vi "Station Detail Main.vi"(8 "error in (no error)":errorcluster, 11 "BarcodeScan in":refnum<class "BarcodeScan.lvclass">) -> (0 "error out":errorcluster, 2 "Station Out":T1=enum."ImformOut", 3 "BarcodeScan out":refnum<class "BarcodeScan.lvclass">)   [LabVIEW 2019, in "BarcodeScan.lvclass"]
uses:
  BarcodeScan.lvclass
  Ctrl/Station Action.ctl
  Ctrl/ProjectStepSelect.ctl
  Ctl/BarcodeStep.ctl
  Ctrl/Auto Inspection Station Name2.ctl
  Ctrl/Auto Inspection Data Name.ctl
  Ctl/Board Scan IO.ctl
  Ctrl/ModbusCmd.ctl
  Ctrl/Table Save.ctl
  Ctrl/MeasureDisplayTab.ctl
  LLB/Commonly VI/Main Glb.vi
  Global/Process Global.vi
  LLB/Commonly VI.lvlib
  LineScan/LineScan.lvclass
panel:
  out "Read Index Data":string
  in  "AddTable 6":string[][](table)=[["Tray Barcode", ""], ["PCBA BARCODE", ""], ["硬體(Tool初始化)", ""], ["company(Tool初始化)", ""], ["耗電流 uA(電流表)", ""], ["電池負載電壓", ""], ["晶片ID(Tool FORMAT)", ""], ["雷雕ID(TOOl scan、藍芽接收器)", ""], ["Format(Tool FORMAT)", ""], ["Programe(Tool Programe)", ""], ["MAC(藍芽接收器)", ""], ["ID(藍芽接收器)", ""], ["KPA(藍芽接收器)", ""], ["溫度(藍芽接收器)", ""], ["SENSOR電池電壓(藍芽接收器)", ""], ["RSSI(藍芽接收器)", ""], ["SensorType_315(FSK scan)", ""], ["FSKsnVol_315(FSK scan)", ""], ["FSKscanl_315(FSK scan)", ""], ["P_315(Tool FSK scan)", ""], ["T_315(Tool FSK scan)", ""], ["SensorType_433(ASK scan)", ""], ["ASKsnVol_433(ASK scan)", ""], ["ASKscan_433(ASK scan)", ""], ["P_433(ASK scan)", ""], ["T_433(ASK scan)", ""], ["測高Data", ""]]
  out "Rad In Reg":string
  in  "AddTable 2":string[][](table)=[["PCBA BARCODE", ""], ["硬體(Tool初始化)", ""], ["company(Tool初始化)", ""], ["耗電流 uA(電流表)", ""], ["電池負載電壓", ""], ["晶片ID(Tool FORMAT)", ""], ["雷雕ID(TOOl scan、藍芽接收器)", ""], ["Format(Tool FORMAT)", ""], ["Programe(Tool Programe)", ""], ["MAC(藍芽接收器)", ""], ["ID(藍芽接收器)", ""], ["KPA(藍芽接收器)", ""], ["溫度(藍芽接收器)", ""], ["SENSOR電池電壓(藍芽接收器)", ""], ["RSSI(藍芽接收器)", ""], ["SensorType_315(FSK scan)", ""], ["FSKsnVol_315(FSK scan)", ""], ["FSKscanl_315(FSK scan)", ""], ["P_315(Tool FSK scan)", ""], ["T_315(Tool FSK scan)", ""], ["SensorType_433(ASK scan)", ""], ["ASKsnVol_433(ASK scan)", ""], ["ASKscan_433(ASK scan)", ""], ["P_433(ASK scan)", ""], ["T_433(ASK scan)", ""], ["測高Data", ""]]
  out "Barcode":string
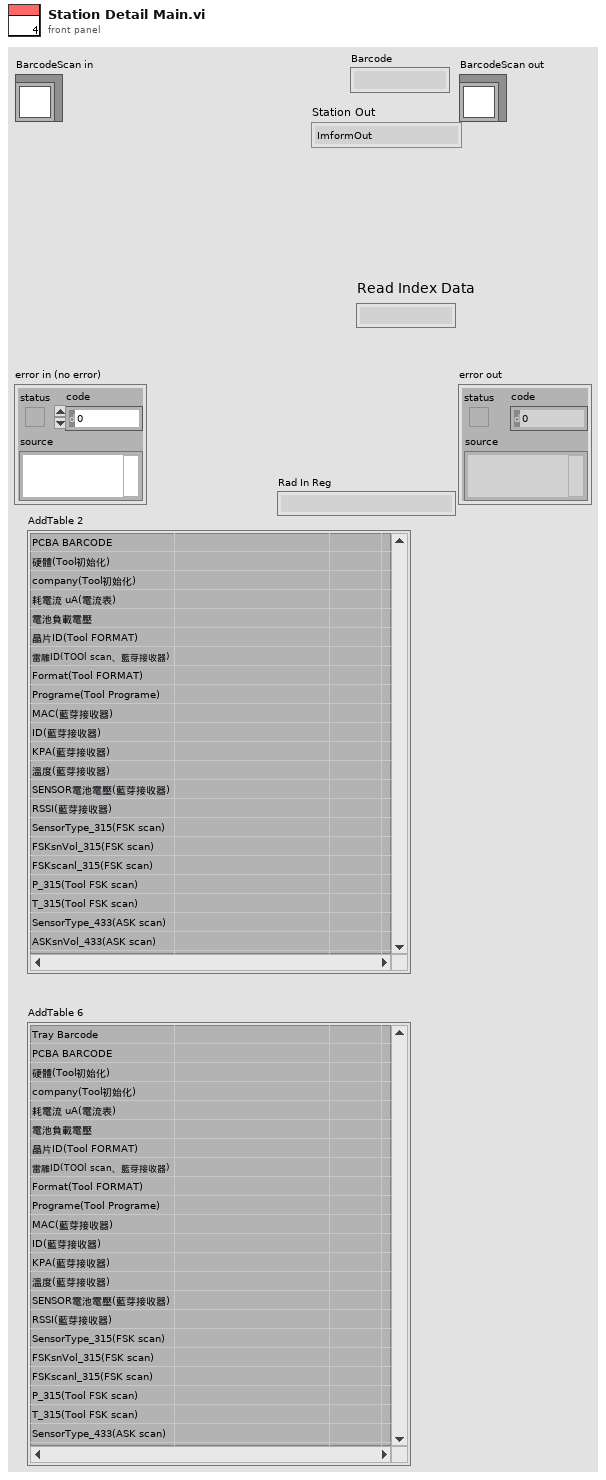
[diagram p1: front panel]
types:
  T1 = typedef "Station Action.ctl" = enum16{"Wait Item In", "Dectect Action", "ImformOut"}
  T2 = typedef "ProjectStepSelect.ctl" = enum16{"ProjectName", "Name", "Initial", "Reset", "Format", "Program1", "Program2", "Scan", "Finish", "MToolWork", "DataCheck", "DataSave", "OutputPLC", "WaitInputS1", "WaitInputOff"}
  T3 = enum16{"initial", "Add", "Write", "Replace", "Delete", "REad"}
  T4 = typedef "Auto Inspection Data Name.ctl" = enum16{"LocalRun", "ItemSN(TimeCode)", "CurrentAction", "Error", "Data", "OKNG", "電壓值", "電壓值判斷", "電流值", "電流值判斷", "Laser1 Data", "Laser2 Data", "Laser OKNG", "StationNO"}
  T5 = typedef "Auto Inspection Station Name2.ctl" = enum16{"S1Barcode", "S2Measure", "S3Measure", "S4Measure", "S5Measure", "S11_LaserCheck", "S8_Vision AI"}
  T6 = cluster{"starting address":u16, "number of inputs":u16, "Sat Coils":bool[], "Holding Registers":u16[]}
  T7 = typedef "ModbusCmd.ctl" = enum16{"Connect", "Disconnect", "Init", "Fetch Basic Objects", "Fetch Input Refisters", "Fetch Discrete Inputs", "Set Coils", "Set Holding Registers", "Write Single Holding", "Exit"}
  T8 = typedef "BarcodeStep.ctl" = enum16{"Initial", "BarcodeScan", "BcdCheck", "BcdCheckOK", "ReadPLCBarcode", "BcdCheckNG", "Merge", "SendPLC_OK", "DataSave", "IOSignal Off", "Finish"}
  T9 = enum16{"載盤條碼比對需求", "載盤條碼比對OK", "載盤條碼比對NG", "S1可讀取訊號"}
  T10 = typedef "Board Scan IO.ctl" = enum16{"S1 Barcode Scan", "回給PLC完成讀取訊號", "S1 載盤條碼比對NG", "S1PLC 條碼可讀取訊號", "S1備用_04", "S1備用_05", "S1備用_06", "S1備用_07", "S1備用_08", "S1 發送條碼完成"}
  T11 = typedef "MeasureDisplayTab.ctl" = enum16{"Tray Barcode", "PCBA BARCODE", "硬體(Tool初始化)", "company(Tool初始化)", "耗電流 uA(電流表)", "電池負載電壓", "晶片ID(Tool FORMAT)", "雷雕ID(TOOl scan、藍芽接收器)", "Format(Tool FORMAT)", "Programe(Tool Programe)", "MAC(藍芽接收器)", "ID(藍芽接收器)", "KPA(藍芽接收器)", "溫度(藍芽接收器)", "SENSOR電池電壓(藍芽接收器)", "RSSI(藍芽接收器)", "SensorType_315(FSK scan)", "FSKsnVol_315(FSK scan)", "FSKscanl_315(FSK scan)", "P_315(FSK scan)", "T_315(FSK scan)", "SensorType_433(ASK scan)", "ASKsnVol_433(ASK scan)", "ASKscan_433(ASK scan)", "P_433(ASK scan)", "T_433(ASK scan)", "測高Data"}
  T12 = typedef "Table Save.ctl" = enum16{"initial", "Add", "Write", "Replace", "Delete", "REad", "RedTable", "Load"}
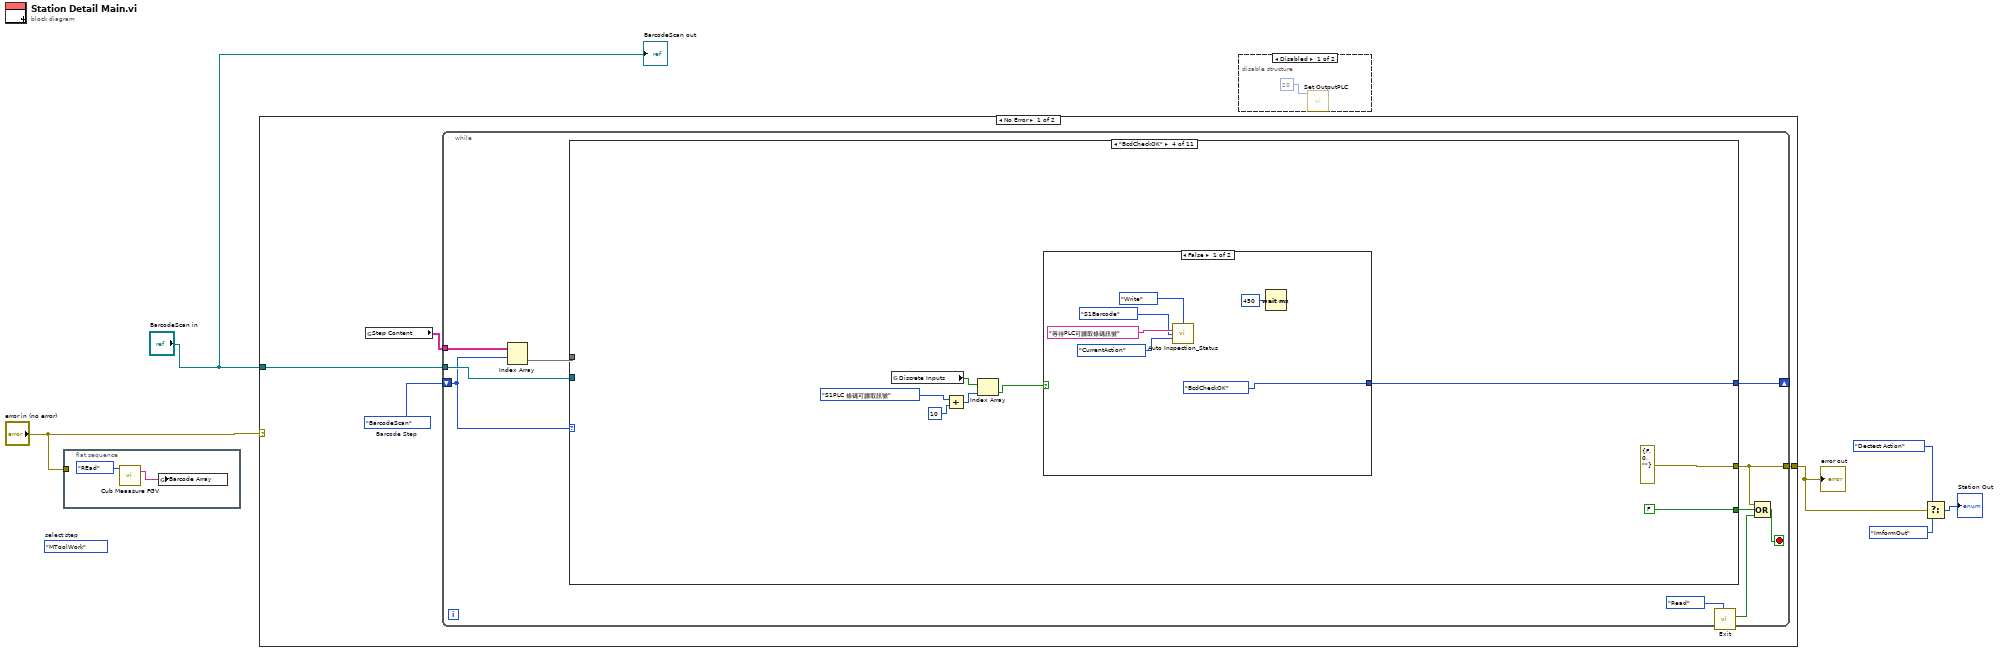
[diagram p0: block diagram]
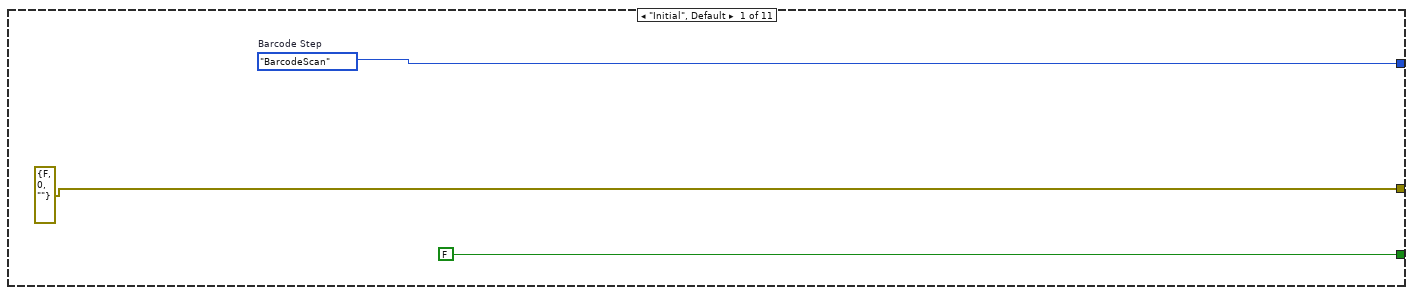
[diagram p3: hidden frame]
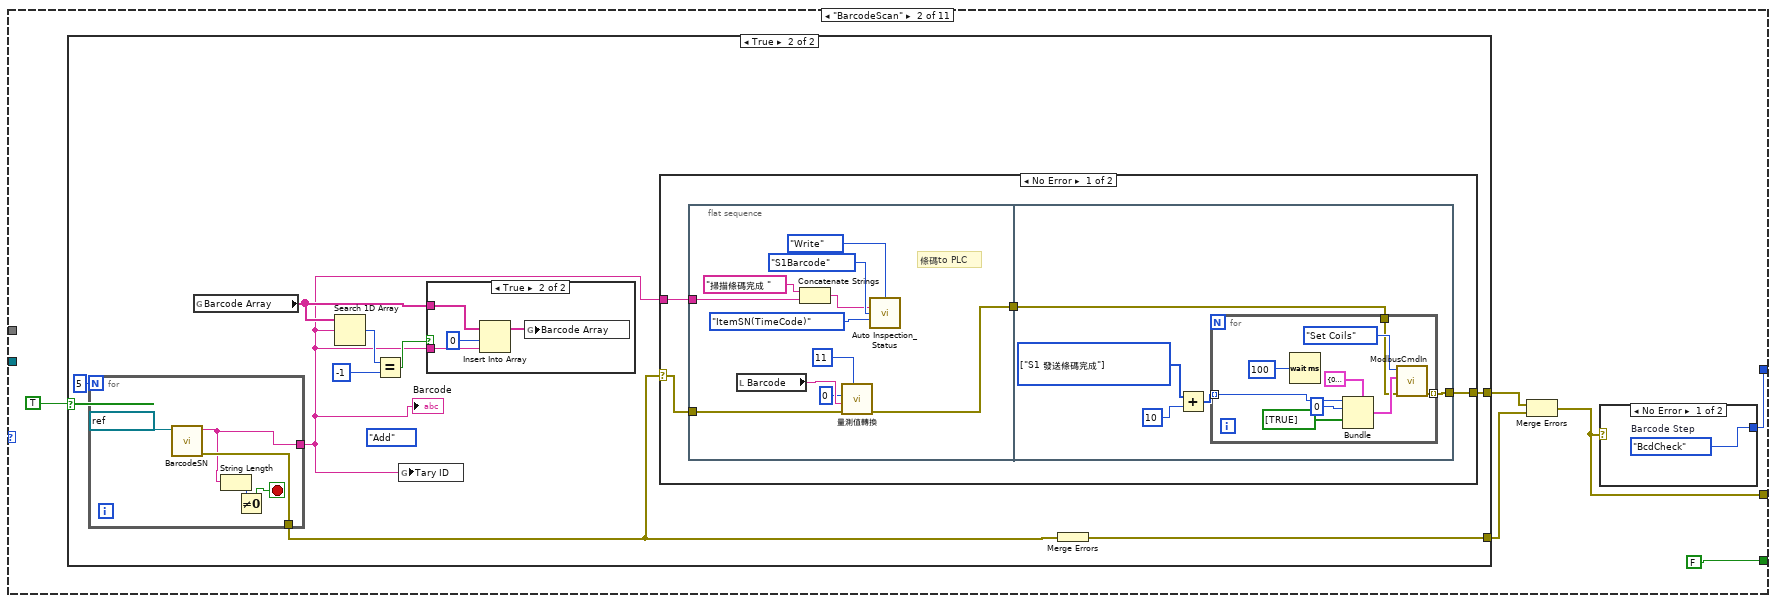
[diagram p4: hidden frame]
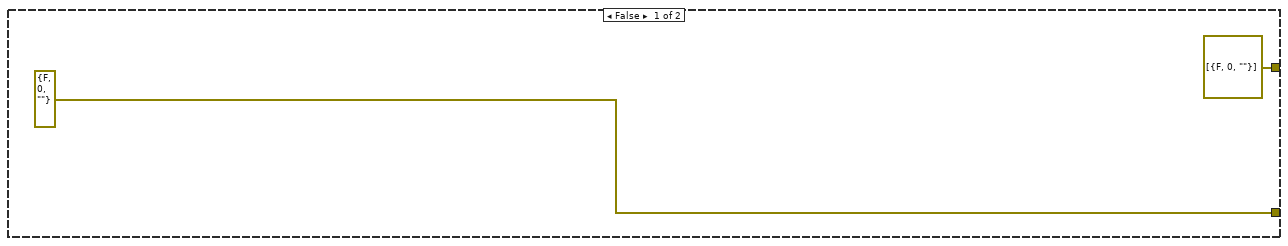
[diagram p5: hidden frame]
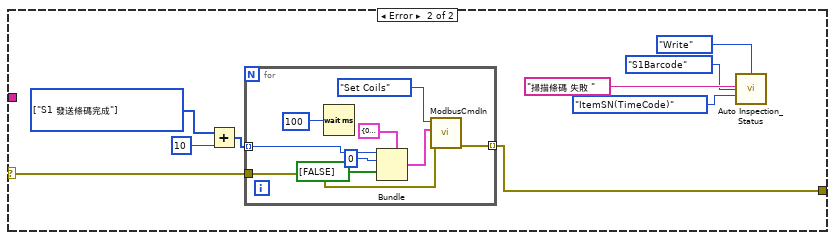
[diagram p6: hidden frame]
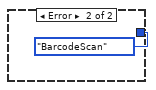
[diagram p8: hidden frame]
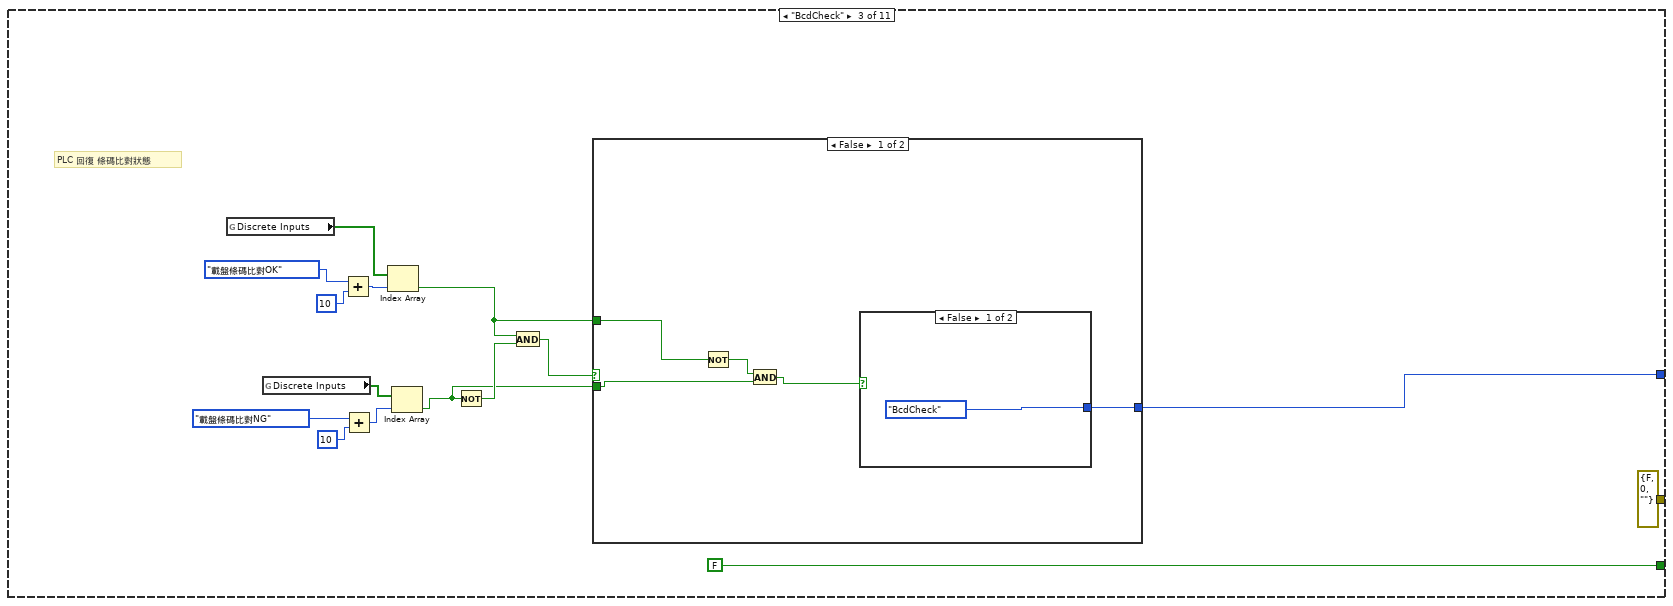
[diagram p9: hidden frame]
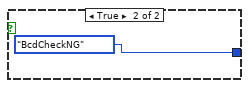
[diagram p10: hidden frame]
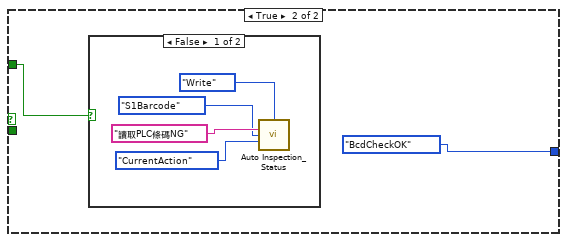
[diagram p11: hidden frame]
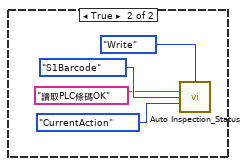
[diagram p12: hidden frame]
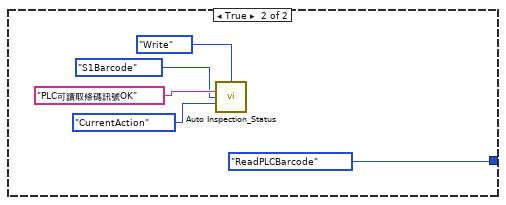
[diagram p13: hidden frame]
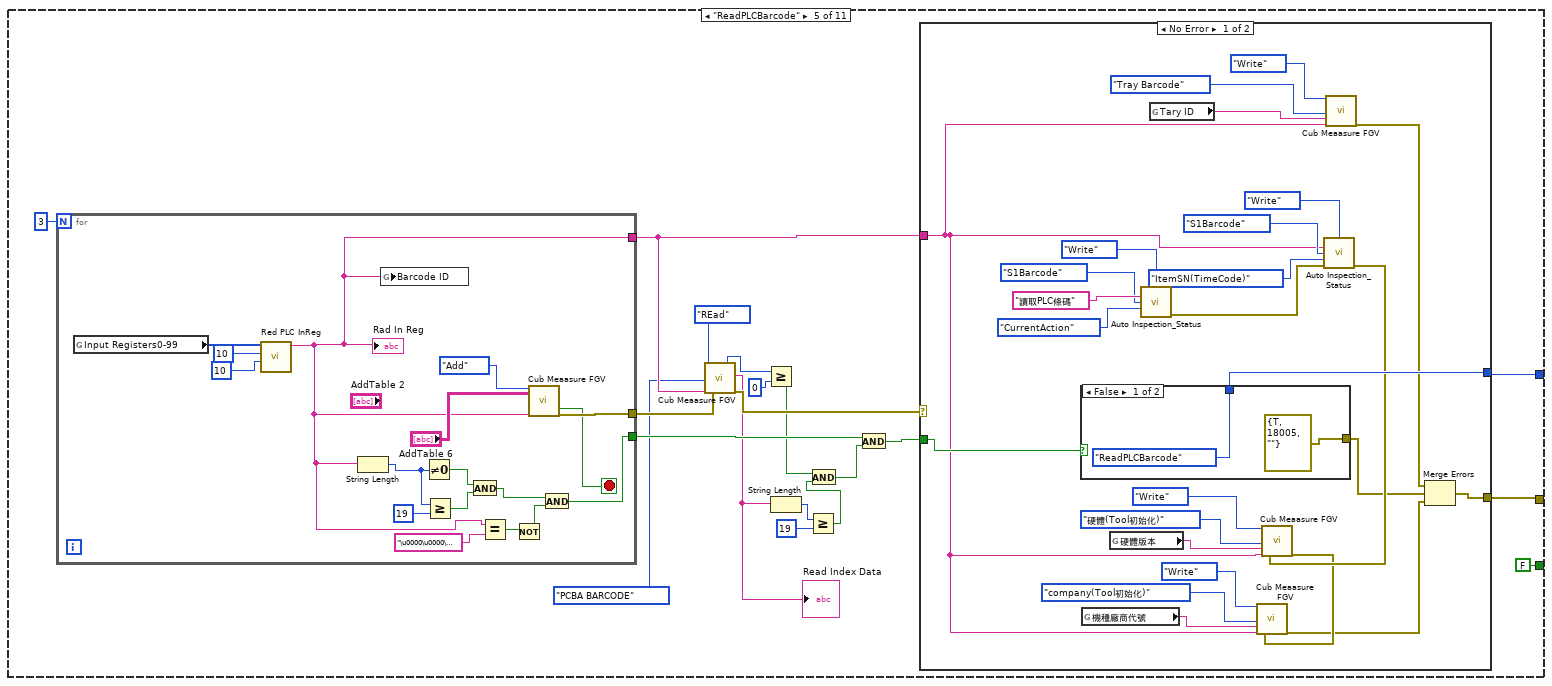
[diagram p14: hidden frame]
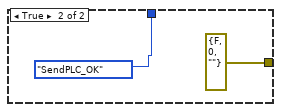
[diagram p15: hidden frame]
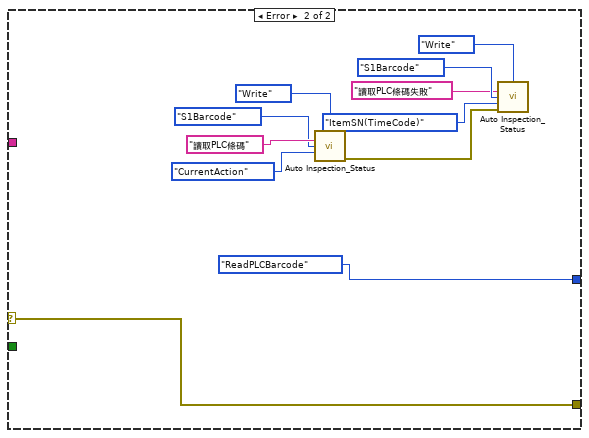
[diagram p16: hidden frame]
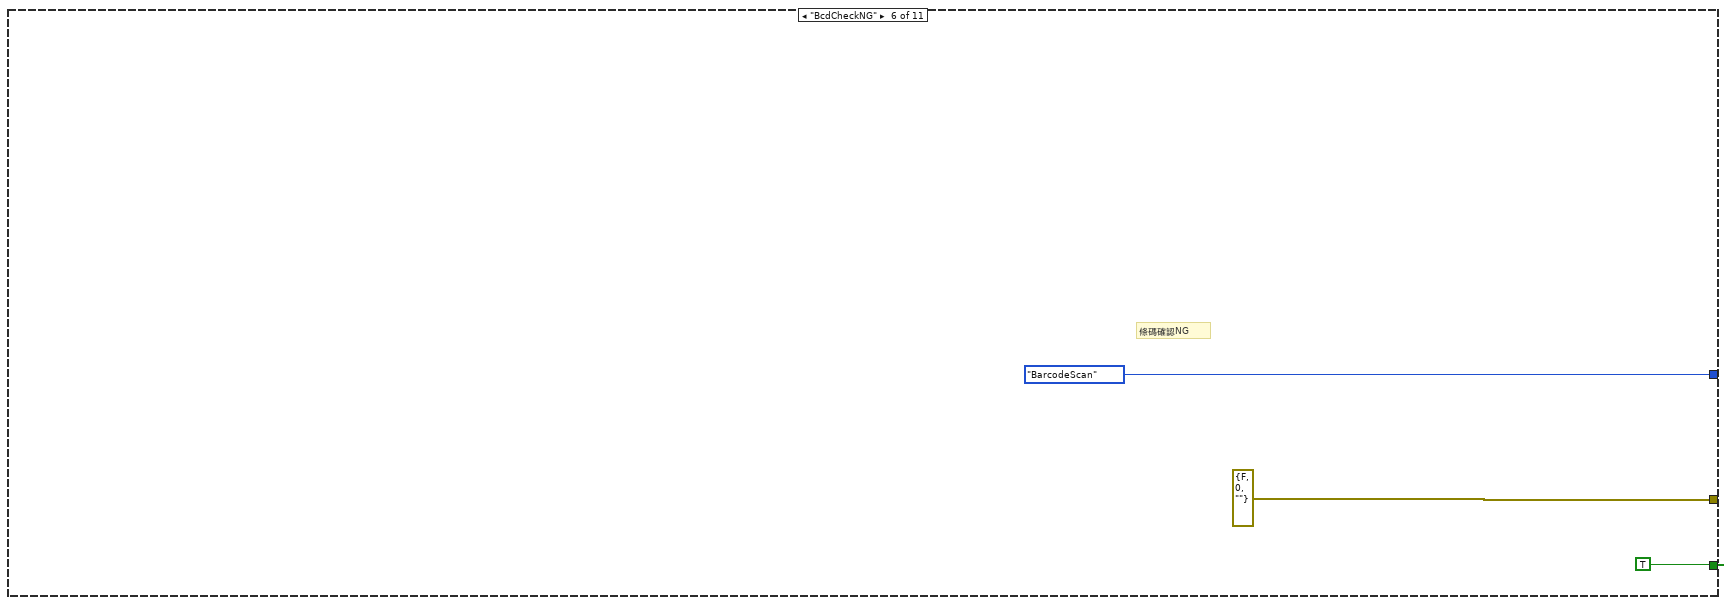
[diagram p17: hidden frame]
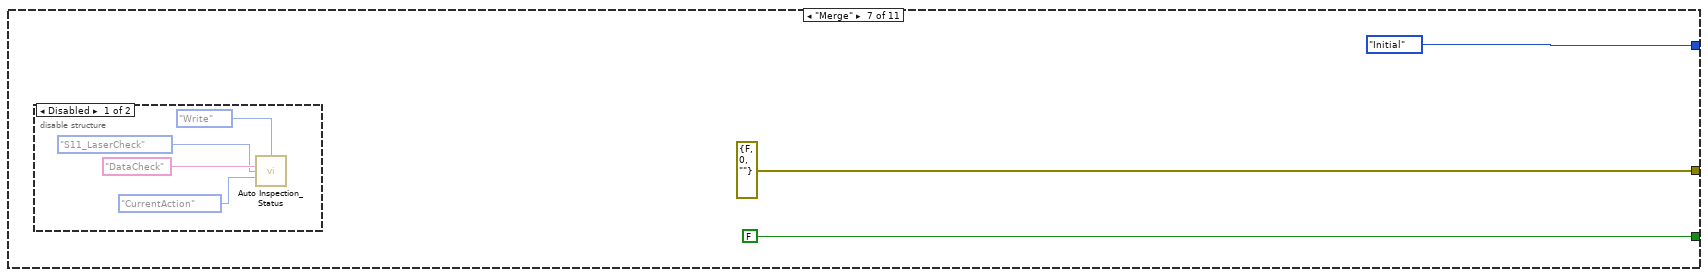
[diagram p18: hidden frame]
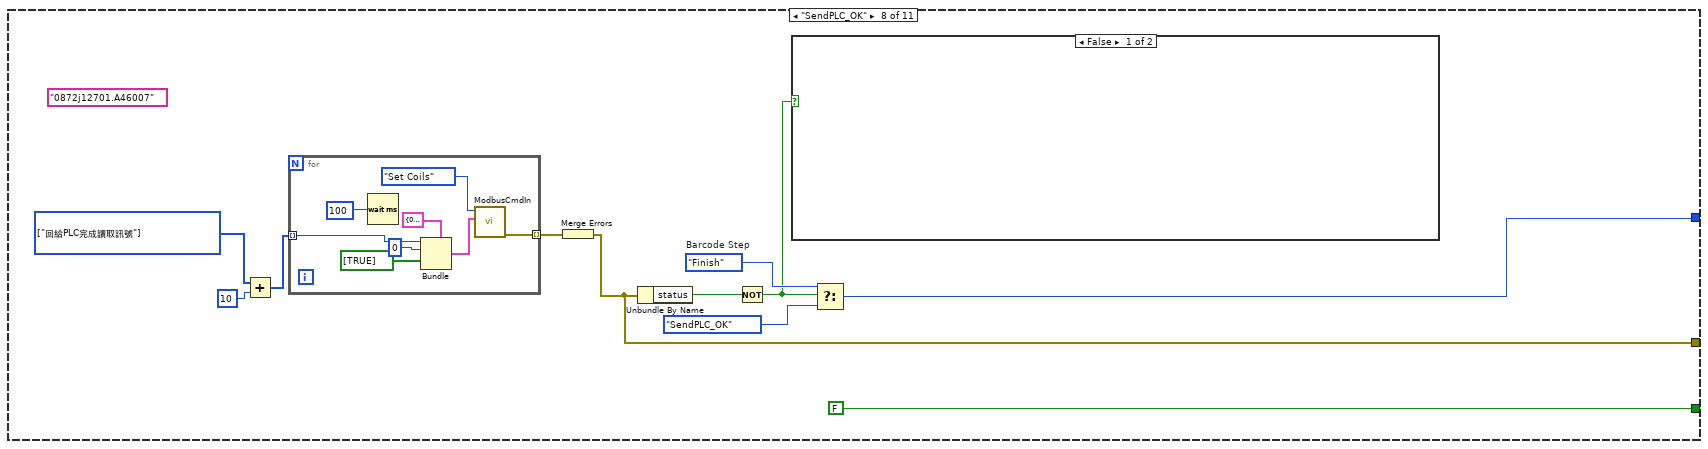
[diagram p20: hidden frame]
diagram:
  (unwired) ProjectStepSelect."MToolWork"  # select step
  n1 = flat-sequence {
    tunnel: "error in (no error)" -> [_]
    frame #0 {
      n2 = call "Cub Meaasure FGV.vi"("Action"=T3."REad" ("Enum")) -> ("Barcode Array"=w8:string[])  [unwired: 11 in, 7 out]
      n3 = global write "Main Glb.vi" "Barcode Array"(w8) -> ()
    }
  }
  n4 = case shown="No Error" "error in (no error)" {
    selector: "error in (no error)" -> [_ w288]
    tunnel: [w12 w288] -> w3
    tunnel: "BarcodeScan in" -> [w11 _]
    frame No Error {
      w9 = BarcodeStep."BarcodeScan"  # Barcode Step
      n5 = global read "Process Global.vi" "Step Content"() -> (w10:string[][])
      n6 = while {
        tunnel: [w17] -> w12
        shift-right: [w22] -> _
        shift-left: w9 -> [w18]
        tunnel: w11 -> [w19]
        tunnel: w10 -> [w20]
        stop <- w16 stop-if-true
        n7 = Index Array(array=w20, index (row)=w18) -> (element=w21:string[])  [unwired: 1 in]
        n8 = case shown="\"BcdCheckOK\"" w18 {
          tunnel: [errorcluster {"status"=FALSE, "code"=0, "source"=""} ("error constant") w26 errorcluster {"status"=FALSE, "code"=0, "source"=""} ("error IO") errorcluster {"status"=FALSE, "code"=0, "source"=""} ("error IO") w169 errorcluster {"status"=FALSE, "code"=0, "source"=""} ("error IO") errorcluster {"status"=FALSE, "code"=0, "source"=""} ("error IO") w239 w259 w267 errorcluster {"status"=FALSE, "code"=0, "source"=""} ("error IO")] -> w17
          tunnel: [w23 w29 w107 w136 w170 BarcodeStep."BarcodeScan" ("Barcode Step") BarcodeStep."Initial" ("Barcode Step") w246 BarcodeStep."IOSignal Off" ("Barcode Step") w268 w285] -> w22
          tunnel: w19 -> [_ _ _ _ _ _ _ _ _ _ _]
          tunnel: w21 -> [_ _ _ _ _ _ _ _ _ _ _]
          tunnel: [FALSE FALSE FALSE FALSE FALSE TRUE FALSE FALSE FALSE FALSE TRUE] -> w15
          frame "Initial", Default {
            w23 = BarcodeStep."BarcodeScan"  # Barcode Step
          }
          frame "BarcodeScan" {
            n9 = case shown="True" TRUE {
              tunnel: [errorcluster {"status"=FALSE, "code"=0, "source"=""} ("error out") w38] -> w27
              tunnel: [errorcluster[] [{"status"=FALSE, "code"=0, "source"=""}] w36] -> w28
              frame False {
              }
              frame True {
                (unwired) T3."Add" ("Enum")
                n10 = for {
                  N: 5 -> [_]
                  tunnel: [w46] -> w37
                  tunnel: [w45] -> w35
                  stop <- w44 stop-if-true
                  n11 = call "BarcodeSN.vi"("VISA resource name"=refnum<visa-resource-name> "COM9") -> ("error out"=w46:errorcluster, "Barcode"=w45:string)  [unwired: 9 in]
                  n12 = String Length(string=w45) -> (length=w43:i32)
                  n13 = Not Equal To 0?(x=w43) -> (x != 0?=w44:bool)
                }
                "Barcode" <- w35
                n14 = global read "Main Glb.vi" "Barcode Array"() -> (w41:string[])
                n15 = Search 1D Array(1D array=w41, element=w35) -> (index of element=w40:i32)  [unwired: 1 in]
                n16 = Equal?(x=w40, y=-1) -> (x = y?=w42:bool)
                n17 = global write "Main Glb.vi" "Tary ID"(w35) -> ()
                n18 = case shown="True" w42 {
                  tunnel: w41 -> [_ w98]
                  tunnel: w35 -> [_ w97]
                  frame False {
                  }
                  frame True {
                    n19 = Insert Into Array(array=w98, index=0, new element=w97) -> (w95:string[])
                    n20 = global write "Main Glb.vi" "Barcode Array"(w95) -> ()
                  }
                }
                n21 = case shown="No Error" w37 {
                  selector: w37 -> [w51 w81]
                  tunnel: [w49 w80] -> w36
                  tunnel: w35 -> [w48 _]
                  frame No Error {
                    n22 = flat-sequence {
                      tunnel: w51 -> [w56]
                      tunnel: [w55] -> w50
                      tunnel: w48 -> [w53]
                      tunnel: w50 -> [w67]
                      tunnel: [w66] -> w49
                      frame #0 {
                        # "條碼to PLC"
                        n23 = local read "Barcode"() -> (w59:string)
                        n24 = Concatenate Strings("掃描條碼完成 " ("DataIn"), w53) -> (w52:string)
                        n25 = call "量測值轉換.vi"("位數"=11, "error in (no error)"=w56, "input string"=w59, "PLC address"=0) -> ("error out"=w55:errorcluster)  [unwired: 6 in, 1 out]
                        n26 = call "Auto Inspection_Status.vi"("Action"=enum16{"Initial", "Write", "Read"}."Write", "DataIn"=w52, "Station"=Auto_Inspection_Station_Name2."S1Barcode", "Data"=Auto_Inspection_Data_Name."ItemSN(TimeCode)") -> ()  [unwired: 9 in, 3 out]
                      }
                      frame #1 {
                        w65 = T10[] [enum."S1 發送條碼完成"] items=["S1 Barcode Scan", "回給PLC完成讀取訊號", "S1 載盤條碼比對NG", "S1PLC 條碼可讀取訊號", "S1備用_04", "S1備用_05", "S1備用_06", "S1備用_07", "S1備用_08", "S1 發送條碼完成"]
                        n27 = Add(x=w65, y=10) -> (x+y=w63:i32[])
                        n28 = for {
                          tunnel: [w70] -> w66 mode=indexing
                          tunnel: w63 -> [w69] mode=indexing
                          tunnel: w67 -> [w68]
                          n29 = Wait (ms)(milliseconds to wait=100) -> ()  [unwired: 1 out]
                          n30 = Bundle(cluster=T6 {"starting address"=0, "number of inputs"=0, "Sat Coils"=[], "Holding Registers"=[]} ("data"), "starting address"=w69, "number of inputs"=u16 0, "Sat Coils"=bool[] [TRUE]) -> (w73:T6)  [unwired: 1 in]
                          n31 = call "ModbusCmdIn.vi"("error in (no error)"=w68, "data"=w73, "Enum"=ModbusCmd."Set Coils") -> ("error out"=w70:errorcluster)  [unwired: 8 in]
                        }
                      }
                    }
                  }
                  frame Error {
                    w79 = T10[] [enum."S1 發送條碼完成"] items=["S1 Barcode Scan", "回給PLC完成讀取訊號", "S1 載盤條碼比對NG", "S1PLC 條碼可讀取訊號", "S1備用_04", "S1備用_05", "S1備用_06", "S1備用_07", "S1備用_08", "S1 發送條碼完成"]
                    n32 = Add(x=w79, y=10) -> (x+y=w77:i32[])
                    n33 = for {
                      tunnel: [w88] -> w80 mode=indexing
                      tunnel: w77 -> [w87] mode=indexing
                      tunnel: w81 -> [w86]
                      n34 = Wait (ms)(milliseconds to wait=100) -> ()  [unwired: 1 out]
                      n35 = Bundle(cluster=T6 {"starting address"=0, "number of inputs"=0, "Sat Coils"=[], "Holding Registers"=[]} ("data"), "starting address"=w87, "number of inputs"=u16 0, "Sat Coils"=bool[] [FALSE]) -> (w91:T6)  [unwired: 1 in]
                      n36 = call "ModbusCmdIn.vi"("error in (no error)"=w86, "data"=w91, "Enum"=ModbusCmd."Set Coils") -> ("error out"=w88:errorcluster)  [unwired: 8 in]
                    }
                    n37 = call "Auto Inspection_Status.vi"("Action"=enum16{"Initial", "Write", "Read"}."Write", "DataIn"="掃描條碼 失敗 ", "Station"=Auto_Inspection_Station_Name2."S1Barcode", "Data"=Auto_Inspection_Data_Name."ItemSN(TimeCode)") -> ()  [unwired: 9 in, 3 out]
                  }
                }
                n38 = Merge Errors(w37) -> (w38:errorcluster)
              }
            }
            n39 = Merge Errors(w28, w27) -> (w26:errorcluster)
            n40 = case shown="No Error" w26 {
              tunnel: [w99 BarcodeStep."BarcodeScan" ("Barcode Step")] -> w29
              frame No Error {
                w99 = BarcodeStep."BcdCheck"  # Barcode Step
              }
              frame Error {
              }
            }
          }
          frame "BcdCheck" {
            # "PLC 回復 條碼比對狀態"
            n41 = global read "Main Glb.vi" "Discrete Inputs"() -> (w114:bool[])
            n42 = global read "Main Glb.vi" "Discrete Inputs"() -> (w109:bool[])
            n43 = Add(x=T9."載盤條碼比對OK", y=10) -> (x+y=w112:i32)
            n44 = Add(x=T9."載盤條碼比對NG", y=10) -> (x+y=w111:i32)
            n45 = Index Array(array=w114, index=w112) -> (element=w105:bool)
            n46 = Index Array(array=w109, index=w111) -> (element=w104:bool)
            n47 = Not(x=w104) -> (.not. x?=w108:bool)
            n48 = And(x=w105, y=w108) -> (x .and. y?=w106:bool)
            n49 = case shown="False" w106 {
              tunnel: [w116 BarcodeStep."BcdCheckOK" ("Barcode Step")] -> w107
              tunnel: w105 -> [w120 w123]
              tunnel: w104 -> [w118 _]
              frame False {
                n50 = Not(x=w120) -> (.not. x?=w119:bool)
                n51 = And(x=w119, y=w118) -> (x .and. y?=w117:bool)
                n52 = case shown="False" w117 {
                  tunnel: [BarcodeStep."BcdCheck" ("Barcode Step") BarcodeStep."BcdCheckNG" ("Barcode Step")] -> w116
                  frame False {
                  }
                  frame True {
                  }
                }
              }
              frame True {
                n53 = case shown="False" w123 {
                  frame False {
                    n54 = call "Auto Inspection_Status.vi"("Action"=enum16{"Initial", "Write", "Read"}."Write", "DataIn"="讀取PLC條碼NG", "Station"=Auto_Inspection_Station_Name2."S1Barcode", "Data"=Auto_Inspection_Data_Name."CurrentAction") -> ()  [unwired: 9 in, 3 out]
                  }
                  frame True {
                    n55 = call "Auto Inspection_Status.vi"("Action"=enum16{"Initial", "Write", "Read"}."Write", "DataIn"="讀取PLC條碼OK", "Station"=Auto_Inspection_Station_Name2."S1Barcode", "Data"=Auto_Inspection_Data_Name."CurrentAction") -> ()  [unwired: 9 in, 3 out]
                  }
                }
              }
            }
          }
          frame "BcdCheckOK" {
            n56 = global read "Main Glb.vi" "Discrete Inputs"() -> (w140:bool[])
            n57 = Add(x=Board_Scan_IO."S1PLC 條碼可讀取訊號" ("Enum"), y=10) -> (x+y=w138:i32)
            n58 = Index Array(array=w140, index=w138) -> (element=w135:bool)
            n59 = case shown="False" w135 {
              tunnel: [BarcodeStep."BcdCheckOK" ("Barcode Step") BarcodeStep."ReadPLCBarcode" ("Barcode Step")] -> w136
              frame False {
                n60 = call "Auto Inspection_Status.vi"("Action"=enum16{"Initial", "Write", "Read"}."Write", "DataIn"="等待PLC可讀取條碼訊號", "Station"=Auto_Inspection_Station_Name2."S1Barcode", "Data"=Auto_Inspection_Data_Name."CurrentAction") -> ()  [unwired: 9 in, 3 out]
                n61 = Wait (ms)(milliseconds to wait=u32 450) -> ()  [unwired: 1 out]
              }
              frame True {
                n62 = call "Auto Inspection_Status.vi"("Action"=enum16{"Initial", "Write", "Read"}."Write", "DataIn"="PLC可讀取條碼訊號OK", "Station"=Auto_Inspection_Station_Name2."S1Barcode", "Data"=Auto_Inspection_Data_Name."CurrentAction") -> ()  [unwired: 9 in, 3 out]
              }
            }
          }
          frame "ReadPLCBarcode" {
            n63 = for {
              N: 3 -> [_]
              tunnel: [w171] -> w166
              tunnel: [w183] -> w160
              tunnel: [w176] -> w165
              stop <- w182 stop-if-true
              n64 = global read "Main Glb.vi" "Input Registers0-99"() -> (w187:u16[])
              n65 = call "Red PLC InReg.vi"("length"=10, "index"=10, "Input Registers Arr"=w187) -> ("Rad In Reg"=w176:string)  [unwired: 7 in, 1 out]
              "Rad In Reg" <- w176
              n66 = String Length(string=w176) -> (length=w180:i32)
              n67 = global write "Main Glb.vi" "Barcode ID"(w176) -> ()
              n68 = Not Equal To 0?(x=w180) -> (x != 0?=w178:bool)
              n69 = Greater Or Equal?(x=w180, y=19) -> (x >= y?=w177:bool)
              n70 = And(x=w178, y=w177) -> (x .and. y?=w172:bool)
              n71 = Equal?(x=w176, y="\u0000\u0000\u0000\u0000\u0000\u0000\u0000\u0000\u0000\u0000\u0000\u0000\u0000\u0000\u0000\u0000\u0000\u0000\u0000\u0000") -> (x = y?=w174:bool)
              n72 = Not(x=w174) -> (.not. x?=w173:bool)
              n73 = call "Cub Meaasure FGV.vi"("Action"=T3."Add" ("Enum"), "AddTable 6"="AddTable 6", "SN"=w176) -> ("Barcode重複"=w182:bool, "error out"=w183:errorcluster)  [unwired: 9 in, 6 out]
              n74 = And(x=w172, y=w173) -> (x .and. y?=w171:bool)
            }
            n75 = call "Cub Meaasure FGV.vi"("Action"=Table_Save."REad", "Save Index"=MeasureDisplayTab."PCBA BARCODE", "SN"=w165, "error in (no error)"=w160) -> ("條碼的Index"=w163:i32, "Read Index Data"=w155:string, "error out"=w159:errorcluster)  [unwired: 8 in, 5 out]
            "Read Index Data" <- w155
            n76 = Greater Or Equal?(x=w163, y=0) -> (x >= y?=w157:bool)
            n77 = String Length(string=w155) -> (length=w154:i32)
            n78 = Greater Or Equal?(x=w154, y=19) -> (x >= y?=w152:bool)
            n79 = And(x=w157, y=w152) -> (x .and. y?=w156:bool)
            n80 = And(x=w166, y=w156) -> (x .and. y?=w161:bool)
            n81 = case shown="No Error" w159 {
              selector: w159 -> [_ w227]
              tunnel: [w213 BarcodeStep."ReadPLCBarcode" ("Enum")] -> w170
              tunnel: w161 -> [w204 _]
              tunnel: [w193 w227] -> w169
              tunnel: w165 -> [w190 _]
              frame No Error {
                n82 = case shown="False" w204 {
                  tunnel: [BarcodeStep."ReadPLCBarcode" ("Enum") BarcodeStep."SendPLC_OK" ("Enum")] -> w213
                  tunnel: [errorcluster {"status"=TRUE, "code"=18005, "source"=""} ("error IO") errorcluster {"status"=FALSE, "code"=0, "source"=""} ("error IO")] -> w194
                  frame False {
                  }
                  frame True {
                  }
                }
                n83 = global read "Process Global.vi" "機種廠商代號"() -> (w198:string)
                n84 = global read "Process Global.vi" "硬體版本"() -> (w199:string)
                n85 = call "Auto Inspection_Status.vi"("Action"=enum16{"Initial", "Write", "Read"}."Write", "DataIn"="讀取PLC條碼", "Station"=Auto_Inspection_Station_Name2."S1Barcode", "Data"=Auto_Inspection_Data_Name."CurrentAction") -> ("error out"=w205:errorcluster)  [unwired: 9 in, 2 out]
                n86 = global read "Main Glb.vi" "Tary ID"() -> (w189:string)
                n87 = call "Auto Inspection_Status.vi"("Action"=enum16{"Initial", "Write", "Read"}."Write", "DataIn"=w190, "Station"=Auto_Inspection_Station_Name2."S1Barcode", "Data"=Auto_Inspection_Data_Name."ItemSN(TimeCode)", "error in"=w205) -> ("error out"=w197:errorcluster)  [unwired: 8 in, 2 out]
                n88 = call "Cub Meaasure FGV.vi"("Action"=Table_Save."Write" ("Enum"), "Save Index"=MeasureDisplayTab."硬體(Tool初始化)", "DataIn"=w199, "SN"=w190, "error in (no error)"=w197) -> ("error out"=w196:errorcluster)  [unwired: 7 in, 7 out]
                n89 = call "Cub Meaasure FGV.vi"("Action"=Table_Save."Write" ("Enum"), "Save Index"=MeasureDisplayTab."company(Tool初始化)", "DataIn"=w198, "SN"=w190, "error in (no error)"=w196) -> ("error out"=w195:errorcluster)  [unwired: 7 in, 7 out]
                n90 = call "Cub Meaasure FGV.vi"("Action"=Table_Save."Write" ("Enum"), "Save Index"=MeasureDisplayTab."Tray Barcode", "DataIn"=w189, "SN"=w190) -> ("error out"=w188:errorcluster)  [unwired: 8 in, 7 out]
                n91 = Merge Errors(w188, w194, w195) -> (w193:errorcluster)
              }
              frame Error {
                n92 = call "Auto Inspection_Status.vi"("Action"=enum16{"Initial", "Write", "Read"}."Write", "DataIn"="讀取PLC條碼", "Station"=Auto_Inspection_Station_Name2."S1Barcode", "Data"=Auto_Inspection_Data_Name."CurrentAction") -> ("error out"=w219:errorcluster)  [unwired: 9 in, 2 out]
                n93 = call "Auto Inspection_Status.vi"("Action"=enum16{"Initial", "Write", "Read"}."Write", "DataIn"="讀取PLC條碼失敗", "Station"=Auto_Inspection_Station_Name2."S1Barcode", "Data"=Auto_Inspection_Data_Name."ItemSN(TimeCode)", "error in"=w219) -> ()  [unwired: 8 in, 3 out]
              }
            }
          }
          frame "BcdCheckNG" {
            # "條碼確認NG"
          }
          frame "Merge" {
            n94 = disable-structure shown="Disabled" {
              frame Disabled {
                n95 = call "Auto Inspection_Status.vi"("Action"=enum16{"Initial", "Write", "Read"}."Write", "DataIn"="DataCheck", "Station"=Auto_Inspection_Station_Name2."S11_LaserCheck", "Data"=Auto_Inspection_Data_Name."CurrentAction") -> ()  [unwired: 9 in, 3 out]
              }
              frame Enabled {
              }
            }
          }
          frame "SendPLC_OK" {
            w242 = T10[] [enum."回給PLC完成讀取訊號"] items=["S1 Barcode Scan", "回給PLC完成讀取訊號", "S1 載盤條碼比對NG", "S1PLC 條碼可讀取訊號", "S1備用_04", "S1備用_05", "S1備用_06", "S1備用_07", "S1備用_08", "S1 發送條碼完成"]
            w247 = BarcodeStep."Finish"  # Barcode Step
            (unwired) "0872j12701.A46007" ("String Input")
            n96 = Add(x=w242, y=10) -> (x+y=w241:i32[])
            n97 = for {
              tunnel: [w251] -> w240 mode=indexing
              tunnel: w241 -> [w250] mode=indexing
              n98 = Wait (ms)(milliseconds to wait=100) -> ()  [unwired: 1 out]
              n99 = Bundle(cluster=T6 {"starting address"=0, "number of inputs"=0, "Sat Coils"=[], "Holding Registers"=[]} ("data"), "starting address"=w250, "number of inputs"=u16 0, "Sat Coils"=bool[] [TRUE]) -> (w254:T6)  [unwired: 1 in]
              n100 = call "ModbusCmdIn.vi"("data"=w254, "Enum"=ModbusCmd."Set Coils") -> ("error out"=w251:errorcluster)  [unwired: 9 in]
            }
            n101 = Merge Errors(w240) -> (w239:errorcluster)
            n102 = Unbundle By Name(w239) -> ("status"=w248:bool)
            n103 = Not(x=w248) -> (.not. x?=w245:bool)
            n104 = case shown="False" w245 {
              frame False {
              }
              frame True {
              }
            }
            n105 = Select(t=w247, s=w245, f=BarcodeStep."SendPLC_OK" ("Barcode Step")) -> (s? t:f=w246:T8)
          }
          frame "DataSave" {
            # "給PLC訊號"
            n106 = disable-structure shown="Enabled" {
              disable-tunnel: [_ errorcluster {"status"=FALSE, "code"=0, "source"=""} ("error IO")] -> w259
              frame Disabled {
              }
              frame Enabled {
                n107 = local read "Barcode"() -> (w261:string)
                n108 = call "Auto Inspection_Status.vi"("Action"=enum16{"Initial", "Write", "Read"}."Write", "DataIn"=w261, "Station"=Auto_Inspection_Station_Name2."S1Barcode", "Data"=Auto_Inspection_Data_Name."ItemSN(TimeCode)") -> ()  [unwired: 9 in, 3 out]
              }
            }
          }
          frame "IOSignal Off" {
            w274 = T10[] [enum."S1 Barcode Scan"] items=["S1 Barcode Scan", "回給PLC完成讀取訊號", "S1 載盤條碼比對NG", "S1PLC 條碼可讀取訊號", "S1備用_04", "S1備用_05", "S1備用_06", "S1備用_07", "S1備用_08", "S1 發送條碼完成"]
            # "條碼掃描完成"
            n109 = for {
              tunnel: w274 -> [w277] mode=indexing
              tunnel: [w275] -> w273 mode=indexing
              n110 = Wait (ms)(milliseconds to wait=100) -> ()  [unwired: 1 out]
              n111 = Add(x=w277, y=u16 10 ("starting address")) -> (x+y=w284:u16)
              n112 = Bundle(cluster=T6 {"starting address"=0, "number of inputs"=0, "Sat Coils"=[], "Holding Registers"=[]} ("data"), "starting address"=w284, "number of inputs"=u16 0, "Sat Coils"=bool[] [FALSE]) -> (w279:T6)  [unwired: 1 in]
              n113 = call "ModbusCmdIn.vi"("data"=w279, "Enum"=ModbusCmd."Set Coils") -> ("error out"=w275:errorcluster)  [unwired: 9 in]
            }
            n114 = Merge Errors(w273) -> (w267:errorcluster)
            n115 = Unbundle By Name(w267) -> ("status"=w272:bool)
            n116 = Not(x=w272) -> (.not. x?=w271:bool)
            n117 = Select(t=BarcodeStep."Finish" ("Barcode Step"), s=w271, f=BarcodeStep."IOSignal Off" ("Barcode Step")) -> (s? t:f=w268:T8)
          }
          frame "Finish" {
            w285 = BarcodeStep."BarcodeScan"  # Barcode Step
          }
        }
        n118 = call "Exit.vi"("Enum"=enum16{"Initial", "Read", "Write"}."Read") -> ("ExitOut"=w14:bool)  [unwired: 10 in]
        n119 = Compound Arithmetic op=OR(w17, w15, w14) -> (w16:bool)
      }
    }
    frame Error {
    }
  }
  "error out" <- w3
  n120 = disable-structure shown="Disabled" {
    frame Disabled {
      n121 = call "Set OutputPLC.vi"("Address In"=20) -> ()  [unwired: 10 in, 1 out]
    }
    frame Enabled {
    }
  }
  n122 = Select(t=Station_Action."Dectect Action" ("Station Out"), s=w3, f=Station_Action."ImformOut" ("Station Out")) -> (s? t:f=→"Station Out":T1)
  "BarcodeScan out" <- "BarcodeScan in"
